vi "Toolkit - Cluster Control Target.vi"() -> ()   [LabVIEW 2017]
doc: "The target VI for the Toolkit - Cluster Control example. Do NOT modify the contents of this VI. This is needed because alphabetizing within a running VI is not possible."
panel:
  in  "Data":T1
  # "Overview: The target VI for the Toolkit- Cluster Control example\nInstructions:\n1. Do not modify or remove\n\nThis is needed for alphabetizing a cluster constant using VI scripting and the ACE toolkit."
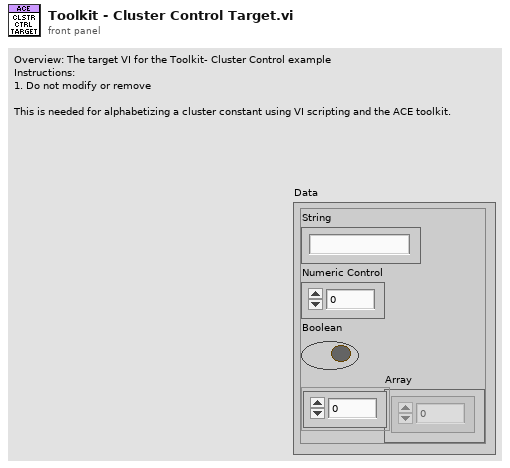
[diagram p1: front panel]
types:
  T1 = cluster{"String":string, "Numeric Control":dbl, "Boolean":bool, "Array":dbl[]}
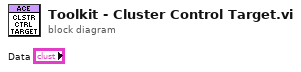
[diagram p0: block diagram]
diagram:
